vi "update time stamp text.vi"() -> ()   [LabVIEW 2021]
panel:
  out "concatenated string":string
  out "date/time string":string
  out "Numeric Text.Text 2":string
  out "Numeric Text.Text":string
  in  "Time Stamp 2":timestamp format="%<%Y-%m-%d %H:%M:%S >T"
  in  "Time Stamp 1":timestamp format="%<%Y-%m-%d %H:%M:%S >T"
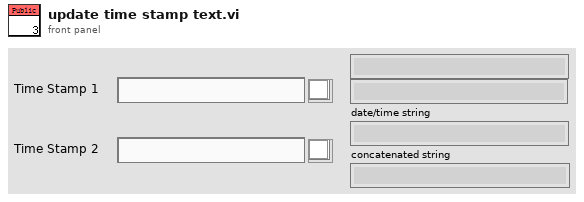
[diagram p1: front panel]
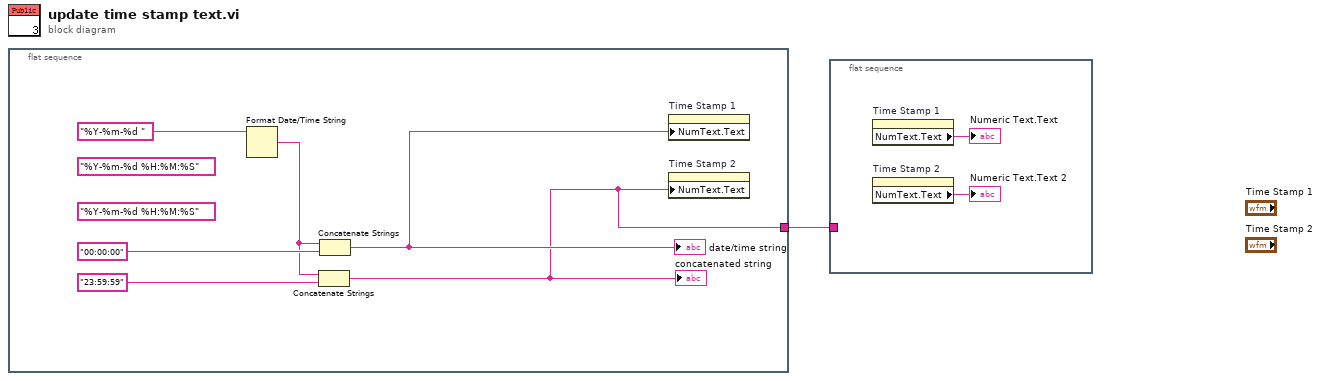
[diagram p0: block diagram]
diagram:
  n1 = flat-sequence {
    tunnel: [w2] -> w1
    frame #0 {
      (unwired) "%Y-%m-%d %H:%M:%S" ("time format string (%c)")
      (unwired) "%Y-%m-%d %H:%M:%S" ("time format string (%c)")
      n2 = Format Date/Time String(time format string (%c)="%Y-%m-%d ") -> (date/time string=w5:string)  [unwired: 2 in]
      n3 = Concatenate Strings(w5, "23:59:59" ("Numeric Text.Text 2")) -> (w2:string)
      "concatenated string" <- w2
      n4 = Concatenate Strings(w5, "00:00:00" ("Numeric Text.Text 2")) -> (w3:string)
      "date/time string" <- w3
      n5 = property on="Time Stamp 1" class="AbsTime (strict)"("NumText.Text"=w3) -> ()  [unwired: 2 in, 2 out]
      n6 = property on="Time Stamp 2" class="AbsTime (strict)"("NumText.Text"=w2) -> ()  [unwired: 2 in, 2 out]
    }
  }
  n7 = flat-sequence {
    tunnel: w1 -> [_]
    frame #0 {
      n8 = property on="Time Stamp 1" class="AbsTime (strict)"() -> ("NumText.Text"=→"Numeric Text.Text":string)  [unwired: 2 in, 2 out]
      n9 = property on="Time Stamp 2" class="AbsTime (strict)"() -> ("NumText.Text"=→"Numeric Text.Text 2":string)  [unwired: 2 in, 2 out]
    }
  }
